vi "Timer Callback 2CPUs.vi"(11 "Timer ID":u8) -> ()   [LabVIEW 2021]
uses:
  <vilib>/myRIO/Express VI/Onboard Devices/LED/LED Express VI.xnode
  <vilib>/myRIO/Instrument Drivers/Onboard IO/DIO/vis/Write.vi
  <vilib>/myRIO/Instrument Drivers/Onboard IO/DIO/DIO.lvlib
  <vilib>/myRIO/Common/Instrument Driver Framework/myRIO v1.0/DIO/typedefs/DIO Channels Enum.ctl
  <vilib>/myRIO/Common/Instrument Driver Framework/myRIO v1.0/DIO/typedefs/DIO Channels List.ctl
  <vilib>/myRIO/Common/Instrument Driver Framework/Utilities/typedefs/Generic FPGA Reference.ctl
  <vilib>/myRIO/Common/Instrument Driver Framework/Utilities/typedefs/myRIO v1.0 Reference.ctl
  <vilib>/myRIO/Common/Instrument Driver Framework/Utilities/typedefs/Hardware Version Enum.ctl
  <vilib>/myRIO/Common/Instrument Driver Framework/Utilities/typedefs/myRIO Generic Hardware Reference.ctl
  <vilib>/myRIO/Instrument Drivers/Onboard IO/DIO/typedefs/DIO Reference.ctl
  <vilib>/myRIO/Instrument Drivers/Onboard IO/DIO/vis/myRIO DIO Open.xnode
  <vilib>/myRIO/Common/Instrument Driver Framework/Utilities/vis/Is FPGA Ref Available.vi
  <vilib>/myRIO/Common/Instrument Driver Framework/myRIO v1.0/DIO/vis/myRIO v1.1 Open DIO.vi
  <vilib>/userdefined/High Color/nirio_resource_hc.ctl
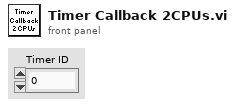
[diagram p1: front panel]
types:
  T1 = typedef "DIO.lvlib/DIO Reference.ctl" = cluster{"myRIO Reference":T2, "DIO Channels List":T6}
  T2 = typedef "myRIO Generic Hardware Reference.ctl" = cluster{"myRIO Model":T3, "myRIO Hardware Reference":T4}
  T3 = typedef "Hardware Version Enum.ctl" = enum16{"Unknown", "myRIO-1900", "myRIO-1950", "roboRIO", "NI ELVIS RIO CM", "ELVIS III"}
  T4 = typedef "myRIO v1.0 Reference.ctl" = cluster{"Generic FPGA Reference":T5, "Allow multiple opens":bool}
  T5 = typedef "Generic FPGA Reference.ctl" = refnum<k20>
  T6 = typedef "DIO Channels List.ctl" = T7[]
  T7 = typedef "DIO Channels Enum.ctl" = enum16{"Not Connected", "C/DIO0", "C/DIO1", "C/DIO2", "C/DIO3", "C/DIO4", "C/DIO5", "C/DIO6", "C/DIO7", "A/DIO0", "A/DIO1", "A/DIO2", "A/DIO3", "A/DIO4", "A/DIO5", "A/DIO6", "A/DIO7", "A/DIO8", "A/DIO9", "A/DIO10", "A/DIO11", "A/DIO12", "A/DIO13", "A/DIO14", "A/DIO15", "A/DIO16", "A/DIO17", "A/DIO18", "A/DIO19", "B/DIO0", "B/DIO1", "B/DIO2", "B/DIO3", "B/DIO4", "B/DIO5", "B/DIO6", "B/DIO7", "B/DIO8", "B/DIO9", "B/DIO10", "B/DIO11", "B/DIO12", "B/DIO13", "B/DIO14", "B/DIO15", "B/DIO16", "B/DIO17", "B/DIO18", "B/DIO19", "LED0", "LED1", "LED2", "LED3", "Button0", "DIO/DIO0", "DIO/DIO1", "DIO/DIO2", "DIO/DIO3", "DIO/DIO4", "DIO/DIO5", "DIO/DIO6", "DIO/DIO7", "DIO/DIO8", "DIO/DIO9", "SPI/CS0", "SPI/CS1", "SPI/CS2", "SPI/CS3", "LED RADIO (Green)", "LED RADIO (Red)", "LED COMM (Green)", "LED COMM (Red)", "LED MODE (Green)", "LED MODE (Red)"}
  T8 = typedef "nirio_resource_hc.ctl" = tag
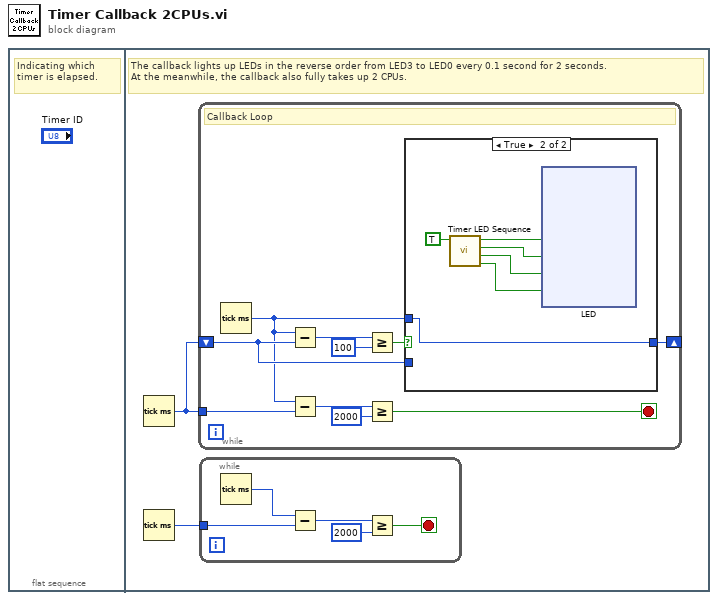
[diagram p0: block diagram]
diagram:
  n1 = flat-sequence {
    frame #0 {
      # "Indicating which timer is elapsed."
    }
    frame #1 {
      # "The callback lights up LEDs in the reverse order from LED3 to LED0 every 0.1 second for 2 seconds.\nAt the meanwhile, the callback also fully takes up 2 CPUs."
      n2 = Tick Count (ms)() -> (millisecond timer value=w2:u32)
      n3 = Tick Count (ms)() -> (millisecond timer value=w1:u32)
      n4 = while {
        tunnel: w2 -> [w17]
        shift-right: [w14] -> _
        shift-left: w2 -> [w10]
        stop <- w8 stop-if-true
        # "Callback Loop"
        n5 = Tick Count (ms)() -> (millisecond timer value=w9:u32)
        n6 = Subtract(x=w9, y=w10) -> (x-y=w13:u32)
        n7 = Subtract(x=w9, y=w17) -> (x-y=w16:u32)
        n8 = Greater Or Equal?(x=w13, y=u32 100) -> (x >= y?=w11:bool)
        n9 = Greater Or Equal?(x=w16, y=u32 2000) -> (x >= y?=w8:bool)
        n10 = case shown="True" w11 {
          tunnel: [w18 w24] -> w14
          tunnel: w9 -> [_ w24]
          tunnel: w10 -> [w18 _]
          frame False {
          }
          frame True {
            n11 = call "Timer LED Sequence.vi"("Reverse?"=TRUE) -> ("LED3"=w20:bool, "LED2"=w21:bool, "LED1"=w22:bool, "LED0"=w23:bool)  [unwired: 7 in]
            n12 = xnode "LED"("LED0"=w23, "LED1"=w22, "LED2"=w21, "LED3"=w20) -> ()  [unwired: 1 in, 1 out]
          }
        }
      }
      n13 = while {
        tunnel: w1 -> [w3]
        stop <- w4 stop-if-true
        n14 = Tick Count (ms)() -> (millisecond timer value=w5:u32)
        n15 = Subtract(x=w5, y=w3) -> (x-y=w6:u32)
        n16 = Greater Or Equal?(x=w6, y=u32 2000) -> (x >= y?=w4:bool)
      }
    }
  }
